vi "字符串数字加1.vi"(1 "OldString":string) -> (0 "NewString":string)   [LabVIEW 2019]
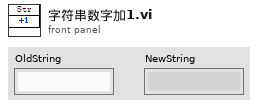
[diagram p1: front panel]
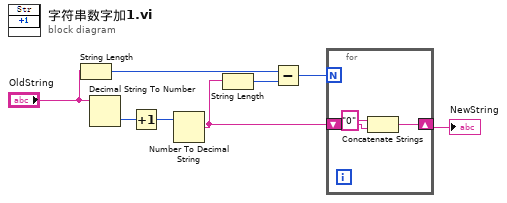
[diagram p0: block diagram]
diagram:
  n1 = String Length(string="OldString") -> (length=w5:i32)
  n2 = Decimal String To Number(string="OldString") -> (number=w7:i32)  [unwired: 2 in, 1 out]
  n3 = Increment(x=w7) -> (x+1=w8:i32)
  n4 = Number To Decimal String(number=w8) -> (decimal integer string=w3:string)  [unwired: 1 in]
  n5 = String Length(string=w3) -> (length=w4:i32)
  n6 = Subtract(x=w5, y=w4) -> (x-y=w2:i32)
  n7 = for {
    N: w2 -> [_]
    shift-right: [w11] -> w1
    shift-left: w3 -> [w10]
    n8 = Concatenate Strings("0" ("string"), w10) -> (w11:string)
  }
  "NewString" <- w1
